vi "WPI_IMU_ADIS16448_OffsetFileName.vi"(1 "PROD_ID":u16, 2 "SERIAL_NUM":u16, 3 "LOT_ID2":u16, 4 "LOT_ID1":u16) -> (0 "RoboRIO Offset Path":path)   [LabVIEW 2015, in "FRC_ADIS16448_IMU.lvlib"]
uses:
  FRC_ADIS16448_IMU.lvlib
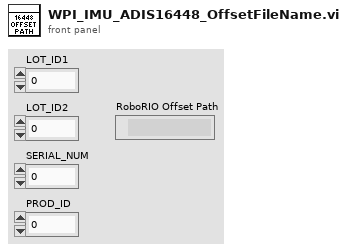
[diagram p1: front panel]
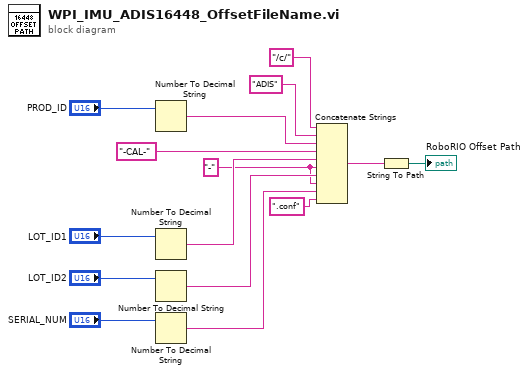
[diagram p0: block diagram]
diagram:
  w12 = "-"
  n1 = Number To Decimal String(number="PROD_ID") -> (decimal integer string=w3:string)  [unwired: 1 in]
  n2 = Number To Decimal String(number="LOT_ID1") -> (decimal integer string=w14:string)  [unwired: 1 in]
  n3 = Number To Decimal String(number="LOT_ID2") -> (decimal integer string=w13:string)  [unwired: 1 in]
  n4 = Number To Decimal String(number="SERIAL_NUM") -> (decimal integer string=w11:string)  [unwired: 1 in]
  n5 = Concatenate Strings("/c/" ("string"), "ADIS" ("string"), w3, "-CAL-", w14, w12, w13, w12, w11, ".conf" ("string")) -> (w6:string)
  n6 = String To Path(string=w6) -> (path=→"RoboRIO Offset Path":path)
